vi "Test Device Thread.vi"() -> ()   [LabVIEW 2015]
uses:
  Control Classes/Base Class/TTLController.lvclass
  Device Classes/Base Class/TTLControlledDevice.lvclass
  Control Classes/Base Class/Trigger.ctl
panel:
  in  "Start 2":T1={"When"="Immediately", "Value"=0.0}
  in  "Stop 2":T1={"When"="After", "Value"=1000.0}
  in  "Send 2":bool
  in  "Start":T1={"When"="Immediately", "Value"=0.0}
  in  "Stop":T1={"When"="After", "Value"=1000.0}
  in  "Send":bool
  in  "stop":bool
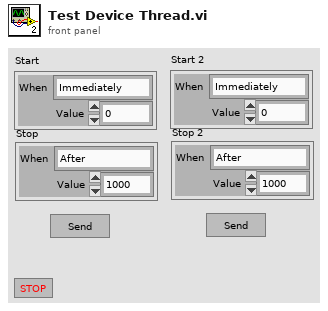
[diagram p1: front panel]
types:
  T1 = typedef "TTLController.lvclass/Trigger.ctl" = cluster{"When":string, "Value":dbl}
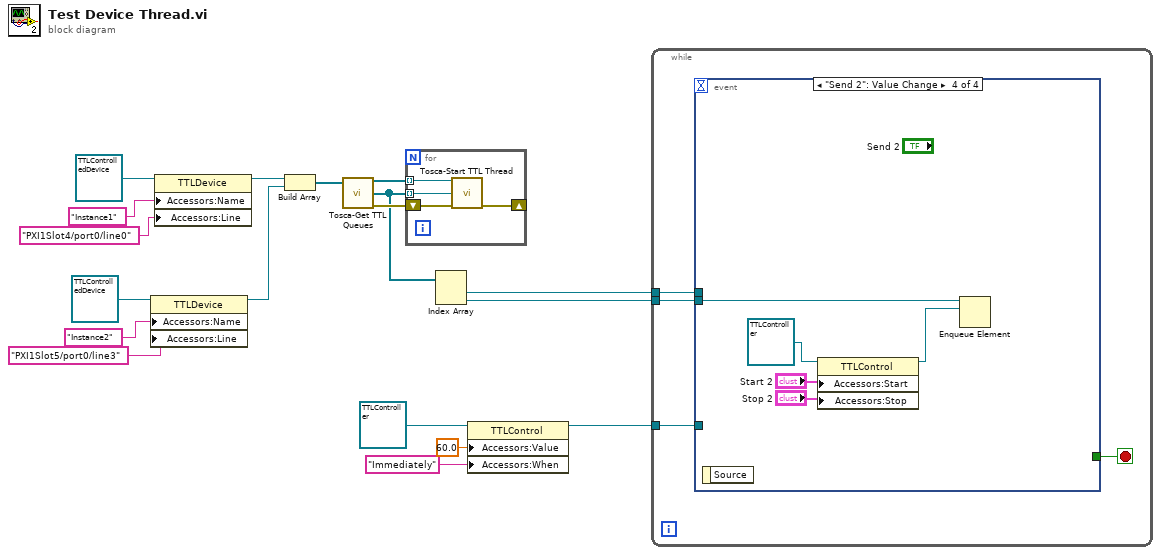
[diagram p0: block diagram]
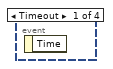
[diagram p2: hidden frame]
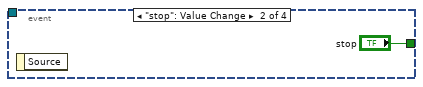
[diagram p3: hidden frame]
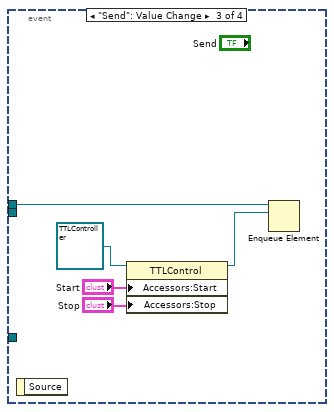
[diagram p4: hidden frame]
diagram:
  n1 = property class="TTLDevice"(reference=refnum<class "TTLControlledDevice.lvclass"> refnum ("TTLDevice"), "Accessors:Name"="Instance2" ("Name"), "Accessors:Line"="PXI1Slot5/port0/line3" ("Line")) -> (reference out=w9:refnum<class "TTLControlledDevice.lvclass">)  [unwired: 1 in, 1 out]
  n2 = property class="TTLDevice"(reference=refnum<class "TTLControlledDevice.lvclass"> refnum ("TTLDevice"), "Accessors:Name"="Instance1" ("Name"), "Accessors:Line"="PXI1Slot4/port0/line0" ("Line")) -> (reference out=w10:refnum<class "TTLControlledDevice.lvclass">)  [unwired: 1 in, 1 out]
  n3 = Build Array(w10, w9) -> (w6:refnum<class "TTLControlledDevice.lvclass">[])
  n4 = call "Tosca-Get TTL Queues.vi"("Devices in"=w6) -> ("Devices out"=w7:refnum<class "TTLControlledDevice.lvclass">[], "Queues"=w5:refnum<queue>[], "error out"=w8:errorcluster)  [unwired: 12 in]
  n5 = for {
    tunnel: w7 -> [w22] mode=indexing
    tunnel: w5 -> [w21] mode=indexing
    shift-right: [w20] -> _
    shift-left: w8 -> [w19]
    n6 = call "Tosca-Start TTL Thread.vi"("TTLDevice"=w22, "Control Queue"=w21, "error in (no error)"=w19) -> ("error out"=w20:errorcluster)  [unwired: 12 in]
  }
  n7 = Index Array(array=w5) -> (element #1=w3:refnum<queue>, element #2=w4:refnum<queue>)  [unwired: 2 in]
  n8 = property class="TTLControl"(reference=refnum<class "TTLController.lvclass"> refnum ("TTLControl"), "Accessors:Value"=60.0 ("Start:Value"), "Accessors:When"="Immediately" ("Start:When")) -> (reference out=w14:refnum<class "TTLController.lvclass">)  [unwired: 1 in, 1 out]
  n9 = while {
    tunnel: w14 -> [w25]
    tunnel: w3 -> [w24]
    tunnel: w4 -> [w23]
    stop <- w26 stop-if-true
    n10 = event shown="[3] \"Send 2\": Value Change" {
      selector: _ -> [_ _ _ _]
      dyn-events: _ -> [_ _ _ _]
      timeout: _ -> [_ _ _ _]
      tunnel: [_ "stop" _ _] -> w26
      tunnel: w25 -> [_ _ _ _]
      tunnel: w24 -> [_ _ w32 _]
      tunnel: w23 -> [_ _ _ w33]
      event Timeout {
        n11 = event-data() -> ()  [unwired: 1 in, 1 out]
      }
      event "stop": Value Change {
        n12 = event-data() -> ()  [unwired: 1 in, 1 out]
      }
      event "Send": Value Change {
        n13 = event-data() -> ()  [unwired: 1 in, 1 out]
        n14 = property class="TTLControl"(reference=refnum<class "TTLController.lvclass"> refnum ("TTLControl"), "Accessors:Start "="Start", "Accessors:Stop "="Stop") -> (reference out=w28:refnum<class "TTLController.lvclass">)  [unwired: 1 in, 1 out]
        n15 = Enqueue Element(queue=w32, element=w28) -> ()  [unwired: 2 in, 3 out]
      }
      event "Send 2": Value Change {
        n16 = event-data() -> ()  [unwired: 1 in, 1 out]
        n17 = property class="TTLControl"(reference=refnum<class "TTLController.lvclass"> refnum ("TTLControl"), "Accessors:Start "="Start 2", "Accessors:Stop "="Stop 2") -> (reference out=w36:refnum<class "TTLController.lvclass">)  [unwired: 1 in, 1 out]
        n18 = Enqueue Element(queue=w33, element=w36) -> ()  [unwired: 2 in, 3 out]
      }
    }
  }
